vi "mainGenerator.vi"() -> ()   [LabVIEW 2017]
uses:
  Control/states.ctl
  <vilib>/ErrorRing/Error Ring.xnode
  <vilib>/measure/NI_MABase.lvlib
panel:
  out "Sinal":waveform(dbl)(graph)={"t0"=timestamp(0 s since 1904-01-01), "dt"=0.0002, "Y"=[]}
  out "Onda":waveform(dbl)(graph)
  in  "Abrir":bool
  in  "Salvar":bool
  in  "Limpa":bool
  in  "Adicionar":bool
  in  "Configurações\n da Onda":T1={"Tipo de forma de onda "=enum."Sine Wave", "Amplitude "=0.0, "Frequencia "=0.0, "Ciclos "=1.0, "Duty Cycle "=0.0, "% Subida "=0.0, "% High "=0.0, "% Descida "=0.0, "Fase "=0.0, "Offset"=0.0, "% Baixo"=0.0, "Amostragem"=0.0} {"Ciclos" min=1.0; "Frequencia" min=0.0}
  in  "Stop Button":bool
  # "Gerador de Sinais"
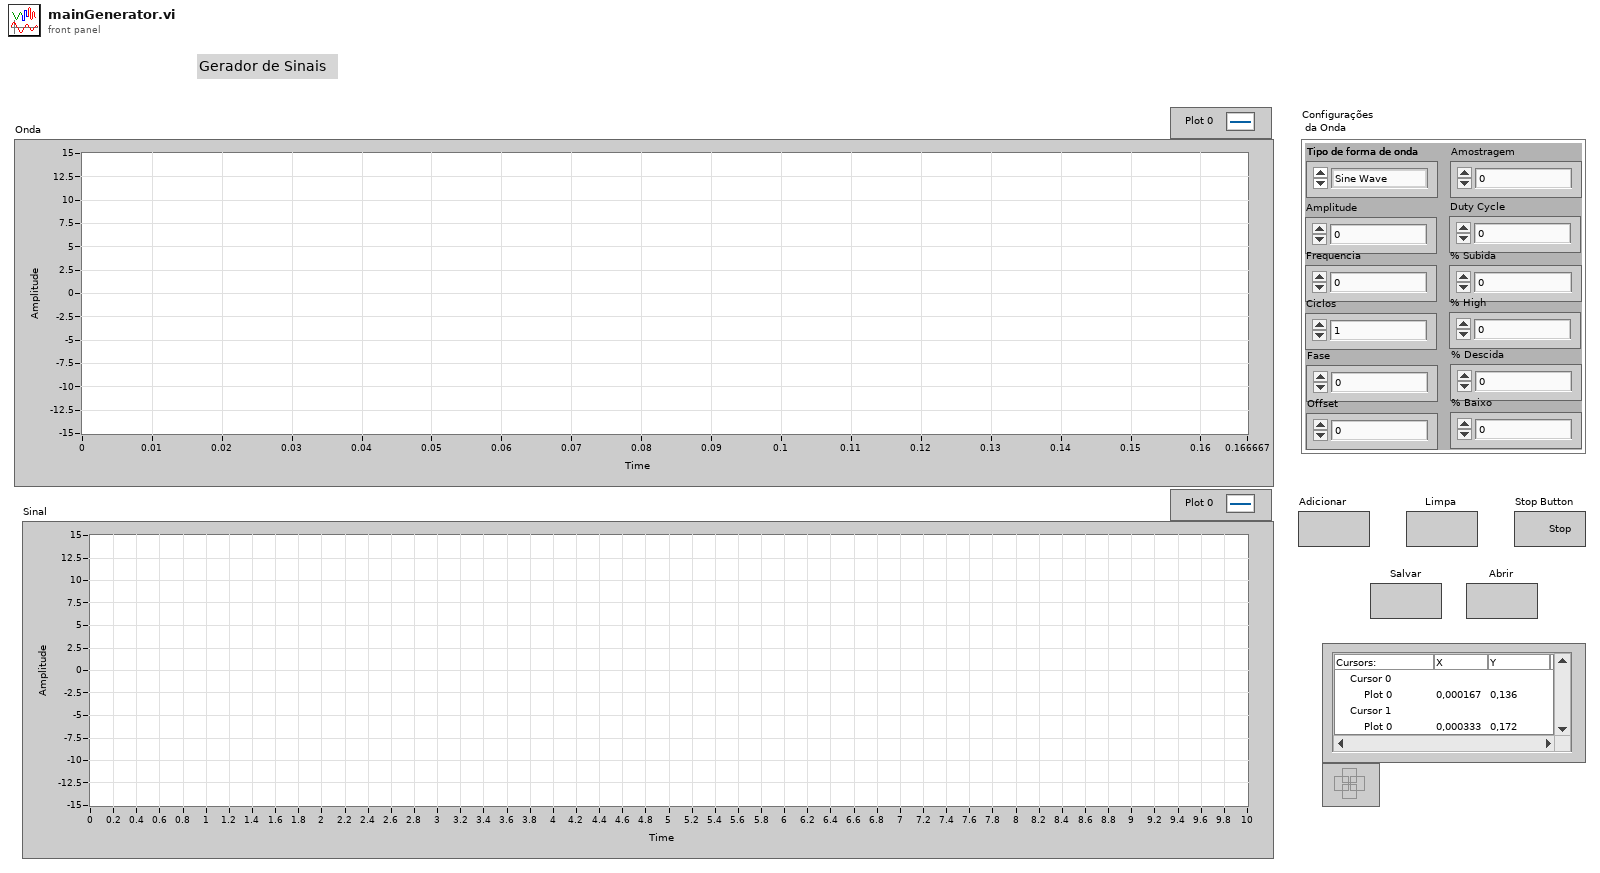
[diagram p1: front panel]
types:
  T1 = cluster{"Tipo de forma de onda ":enum16{"Sine Wave", "Triangle Wave", "Square Wave", "Sawtooth Wave", "Trapezoidal Wave"}, "Amplitude ":dbl, "Frequencia ":dbl, "Ciclos ":dbl, "Duty Cycle ":dbl, "% Subida ":dbl, "% High ":dbl, "% Descida ":dbl, "Fase ":dbl, "Offset":dbl, "% Baixo":dbl, "Amostragem":dbl}
  T2 = typedef "states.ctl" = enum16{"Initialize", "Esperar evento", "Desenha Onda", "Mostra Onda", "Desenha Sinal", "Mostra Sinal", "Clean Graph", "Add", "Remove", "Save", "Open", "Stop"}
  T3 = enum16{"open", "open or create", "create or replace", "create", "open (read-only)"}
  T4 = enum16{"Sine Wave", "Triangle Wave", "Square Wave", "Sawtooth Wave", "Trapezoidal Wave"}
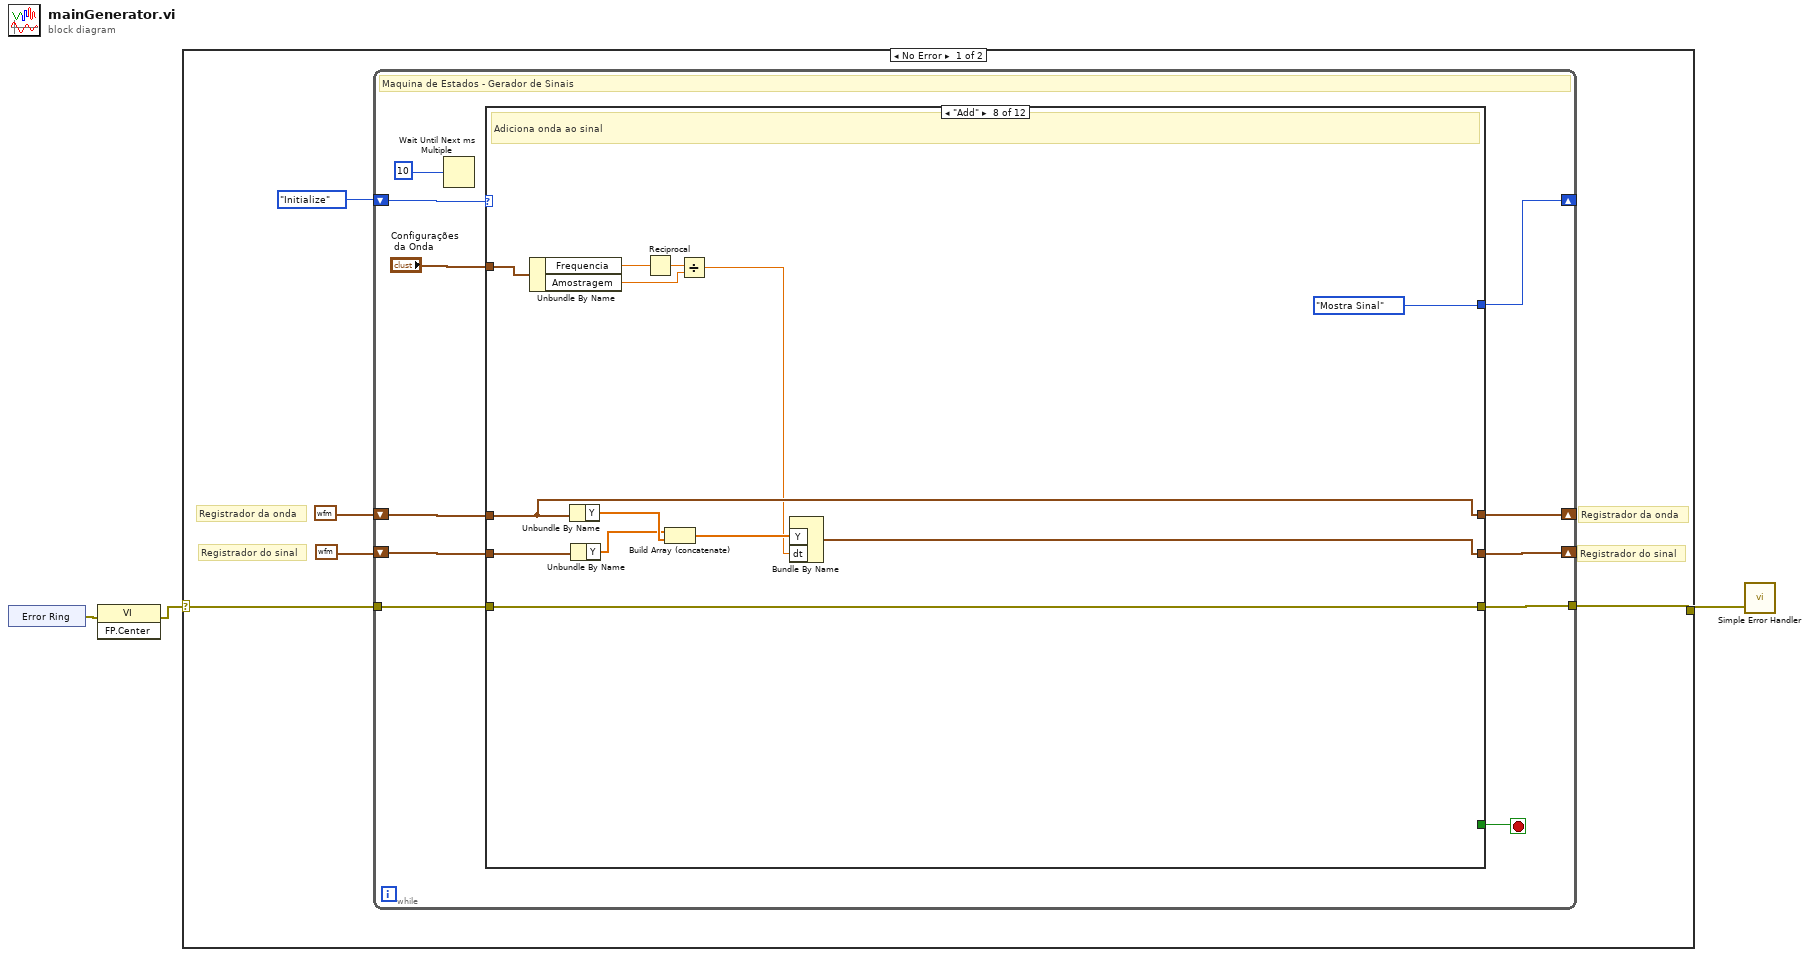
[diagram p0: block diagram]
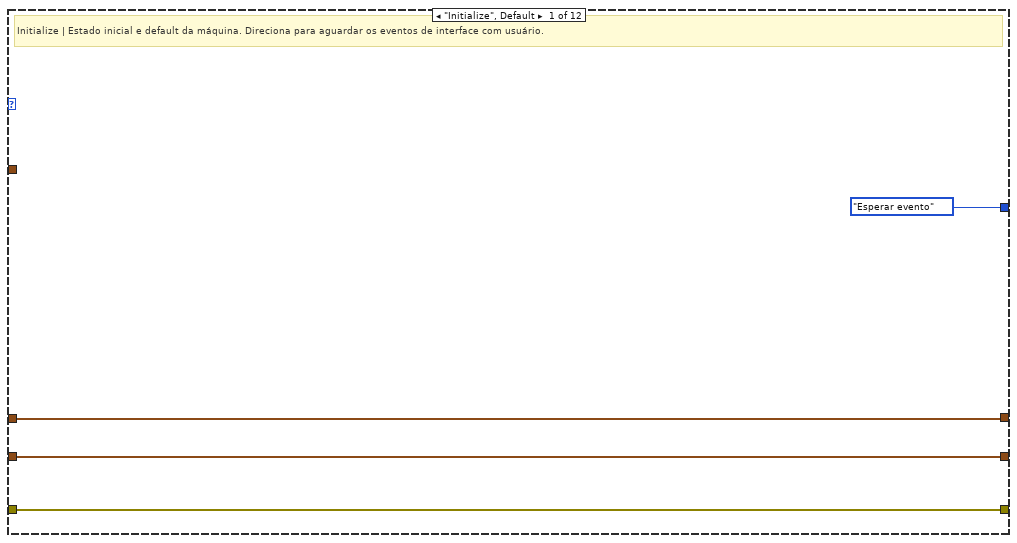
[diagram p2: hidden frame]
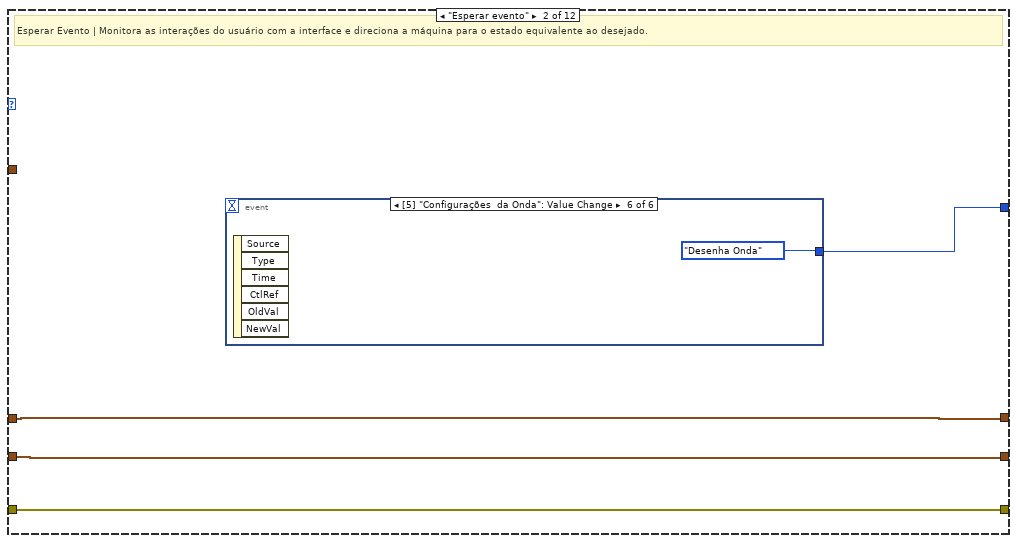
[diagram p3: hidden frame]
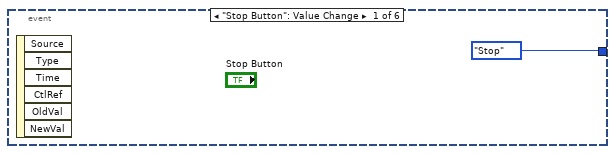
[diagram p4: hidden frame]
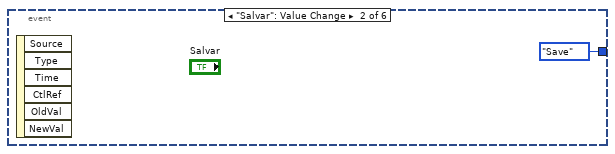
[diagram p5: hidden frame]
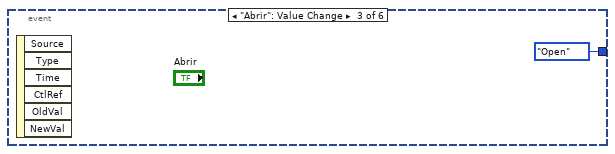
[diagram p6: hidden frame]
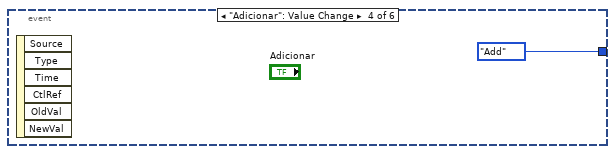
[diagram p7: hidden frame]
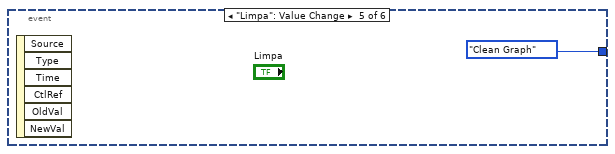
[diagram p8: hidden frame]
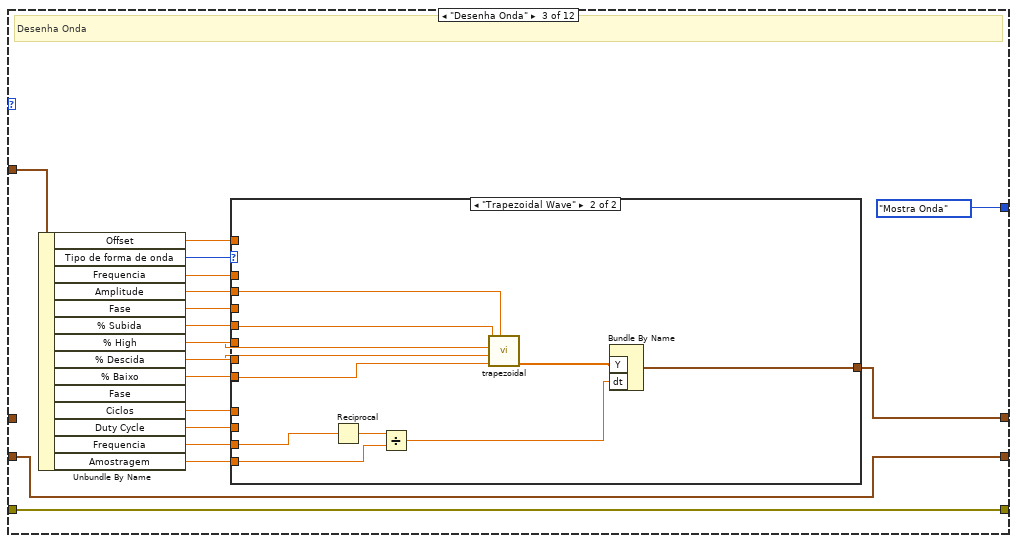
[diagram p9: hidden frame]
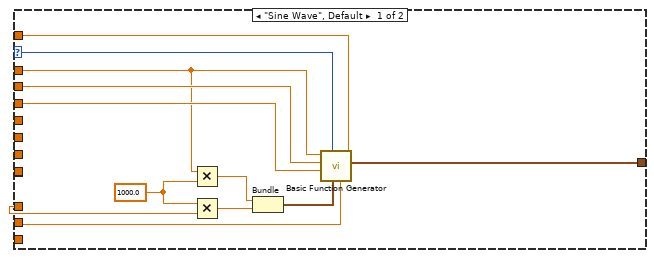
[diagram p10: hidden frame]
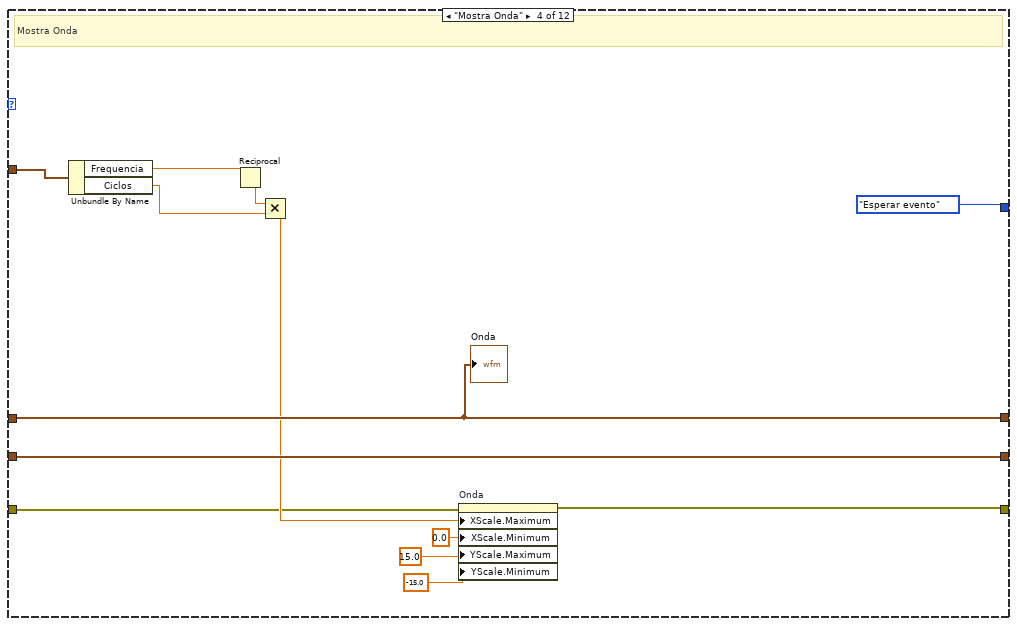
[diagram p11: hidden frame]
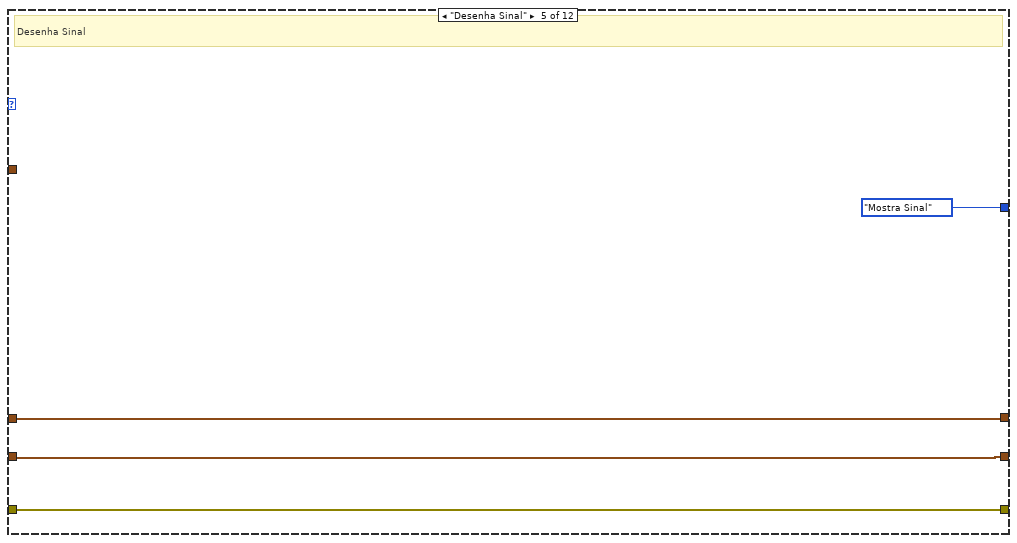
[diagram p12: hidden frame]
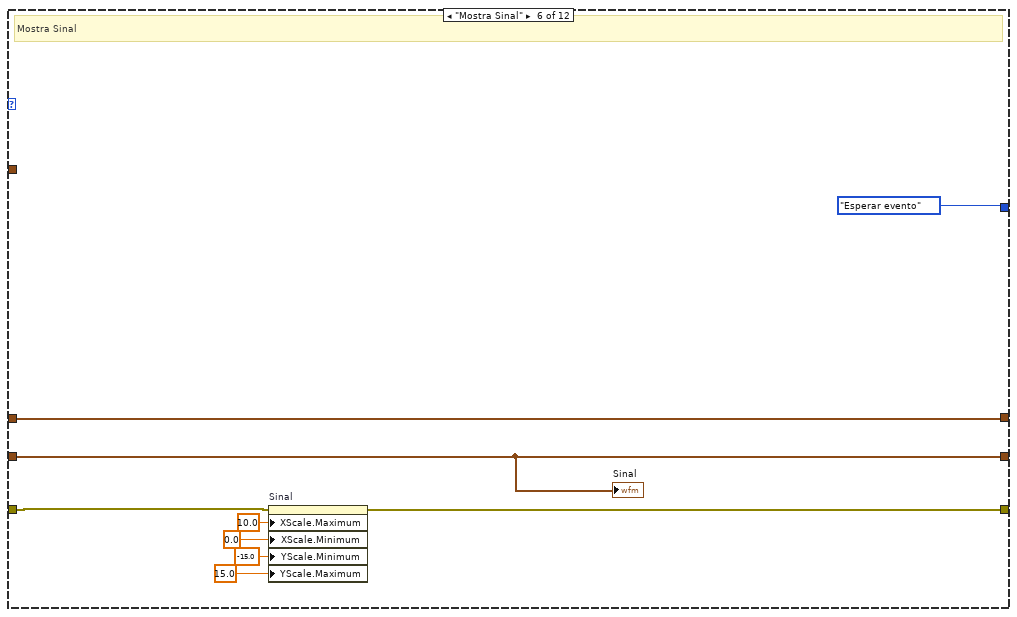
[diagram p13: hidden frame]
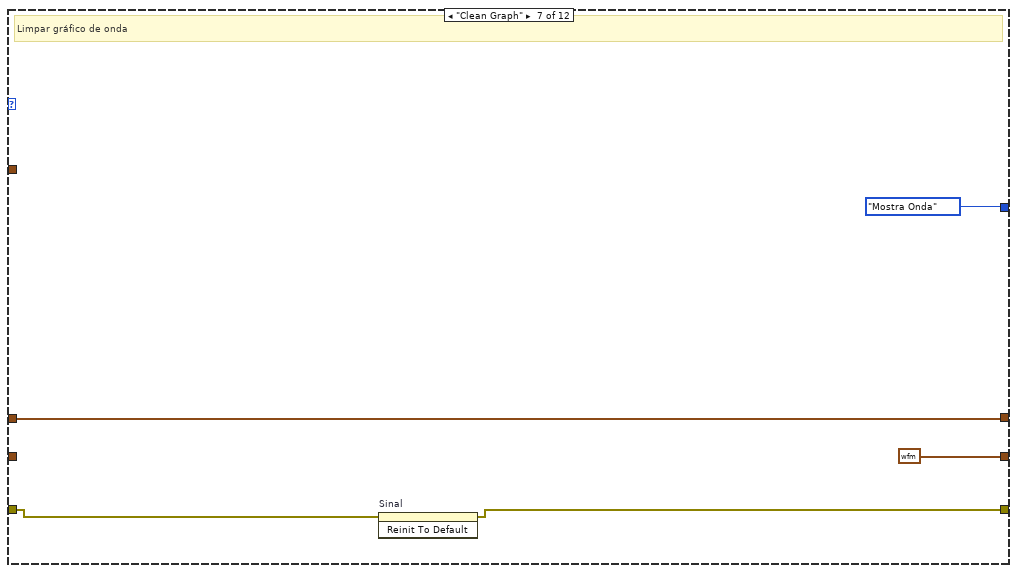
[diagram p14: hidden frame]
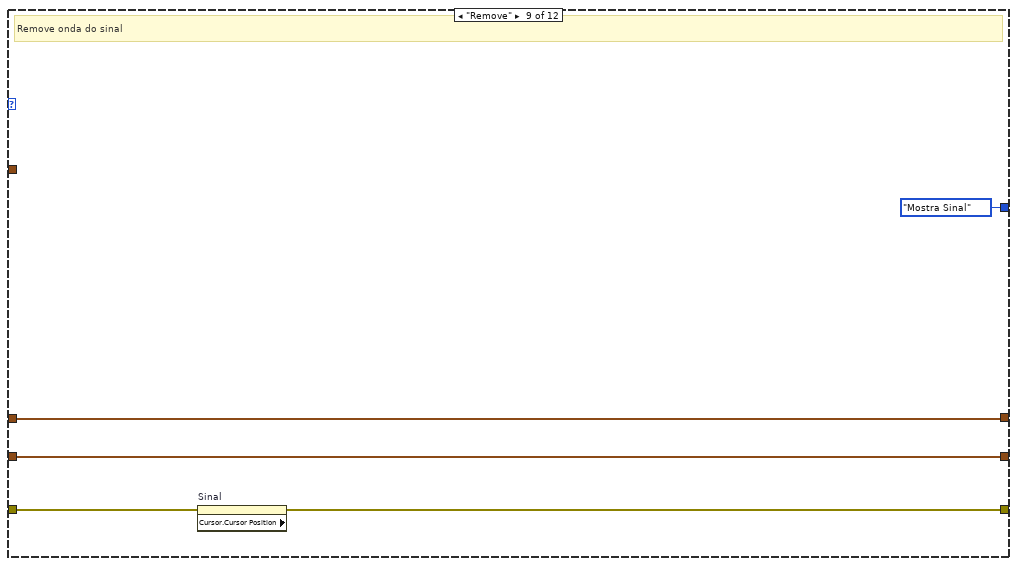
[diagram p15: hidden frame]
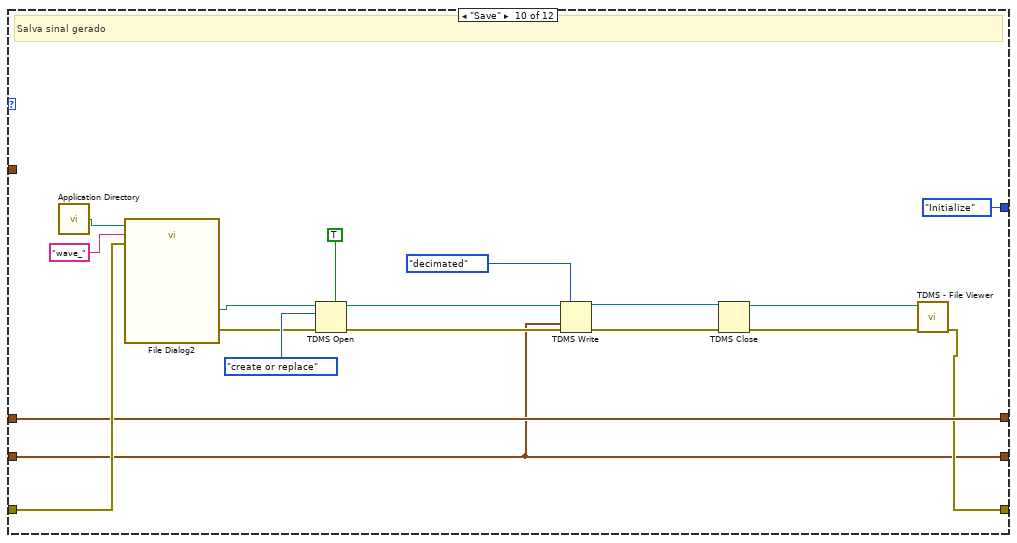
[diagram p16: hidden frame]
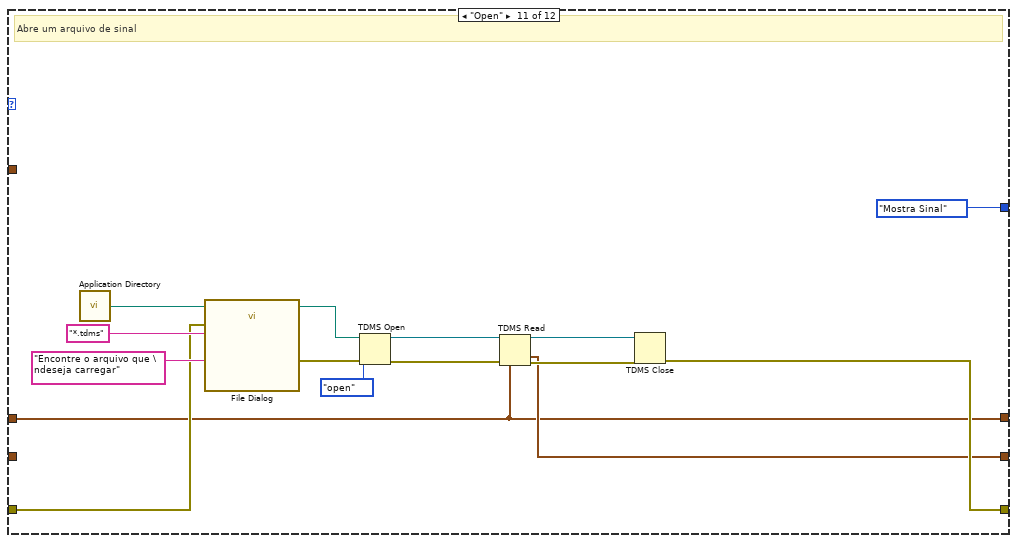
[diagram p17: hidden frame]
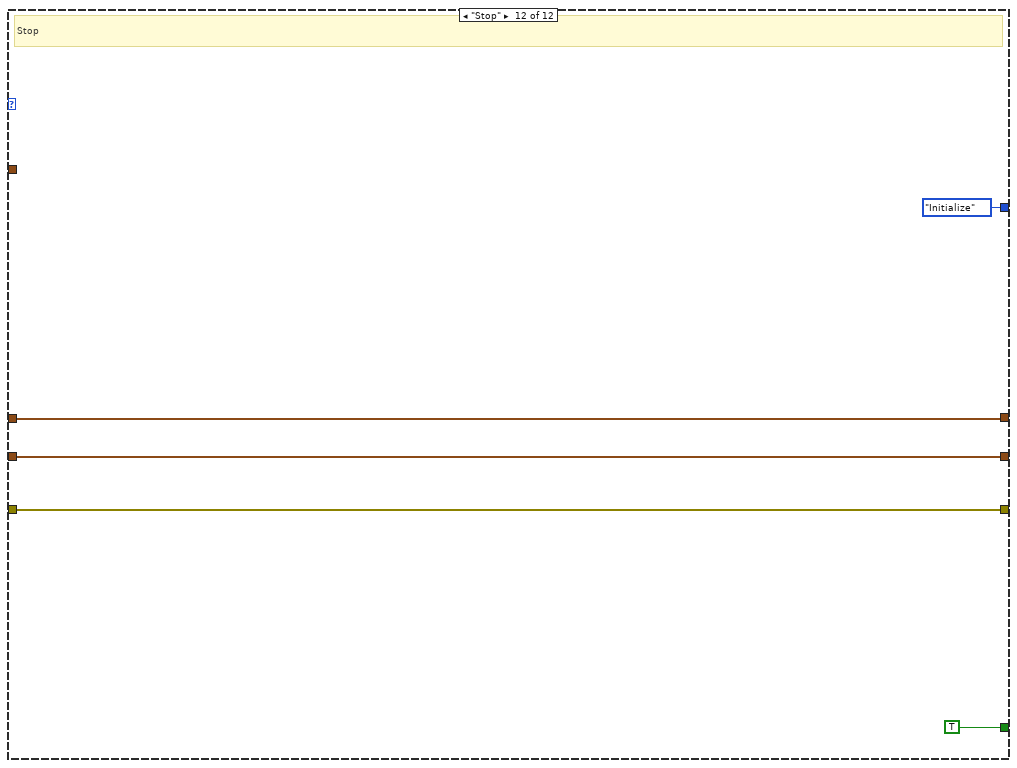
[diagram p18: hidden frame]
diagram:
  n1 = xnode "Error Ring"() -> ("error out"=w3:errorcluster)
  n2 = invoke class="VI" method="FP.Center"(error in=w3) -> (error out=w2:errorcluster)  [unwired: 2 in, 2 out]
  n3 = case shown="No Error" w2 {
    selector: w2 -> [w8 w162]
    tunnel: [w7 w162] -> w1
    frame No Error {
      # "Registrador do sinal"
      # "Registrador da onda"
      # "Registrador do sinal"
      # "Registrador da onda"
      n4 = while {
        shift-right: [w11] -> _
        shift-left: states."Initialize" ("Enum") -> [w12]
        shift-right: [w10] -> _
        shift-left: waveform(dbl) {"t0"=timestamp(0 s since 1904-01-01), "dt"=1.0, "Y"=[]} ("signal out") -> [w13]
        tunnel: [w17] -> w7
        tunnel: w8 -> [w16]
        shift-right: [w14] -> _
        shift-left: waveform(dbl) {"t0"=timestamp(0 s since 1904-01-01), "dt"=1.0, "Y"=[]} ("signal out") -> [w15]
        stop <- w18 stop-if-true
        # "Maquina de Estados - Gerador de Sinais"
        n5 = Wait Until Next ms Multiple(millisecond multiple=u32 10) -> ()  [unwired: 1 out]
        n6 = case shown="\"Add\"" w12 {
          tunnel: [states."Esperar evento" w27 states."Mostra Onda" ("Enum") states."Esperar evento" ("Enum") states."Mostra Sinal" states."Esperar evento" ("Enum") states."Mostra Onda" ("Enum") states."Mostra Sinal" ("Enum") states."Mostra Sinal" ("Enum") states."Initialize" ("Enum") states."Mostra Sinal" ("Enum") states."Initialize" ("Enum")] -> w11
          tunnel: [_ _ _ _ _ _ _ _ _ _ _ TRUE] -> w18
          tunnel: [w21 w24 w37 w83 w90 w100 w104 w108 w122 w128 w142 w161] -> w10
          tunnel: w13 -> [w21 w24 _ w83 w90 w100 w104 w108 w122 w128 w142 w161]
          tunnel: [w23 w26 w35 w75 w91 w92 w101 w107 w119 w125 w146 w160] -> w17
          tunnel: w16 -> [w23 w26 w35 w76 w91 w93 w102 w107 w120 w136 w153 w160]
          tunnel: w15 -> [w22 w25 w41 w87 w88 w98 _ w113 w123 w124 _ w159]
          tunnel: [w22 w25 w41 w87 w88 w98 waveform(dbl) {"t0"=timestamp(0 s since 1904-01-01), "dt"=1.0, "Y"=[]} ("signal out") w109 w123 w124 w143 w159] -> w14
          tunnel: "Configurações\n da Onda" -> [_ _ w39 w85 _ _ _ w117 _ _ _ _]
          frame "Initialize", Default {
            # "Initialize | Estado inicial e default da máquina. Direciona para aguardar os eventos de interface com usuário."
          }
          frame "Esperar evento" {
            # "Esperar Evento | Monitora as interações do usuário com a interface e direciona a máquina para o estado equivalente ao desejado."
            n7 = event shown="[5] \"Configurações  da Onda\": Value Change" {
              selector: _ -> [_ _ _ _ _ _]
              dyn-events: _ -> [_ _ _ _ _ _]
              timeout: _ -> [_ _ _ _ _ _]
              tunnel: [states."Stop" ("Enum") states."Save" ("Enum") states."Open" ("Enum") states."Add" ("Enum") states."Clean Graph" ("Enum") states."Desenha Onda" ("Enum")] -> w27
              event "Stop Button": Value Change {
                n8 = event-data() -> ()  [unwired: 1 in, 6 out]
              }
              event "Salvar": Value Change {
                n9 = event-data() -> ()  [unwired: 1 in, 6 out]
              }
              event "Abrir": Value Change {
                n10 = event-data() -> ()  [unwired: 1 in, 6 out]
              }
              event "Adicionar": Value Change {
                n11 = event-data() -> ()  [unwired: 1 in, 6 out]
              }
              event "Limpa": Value Change {
                n12 = event-data() -> ()  [unwired: 1 in, 6 out]
              }
              event "Configurações\n da Onda": Value Change {
                n13 = event-data() -> ()  [unwired: 1 in, 6 out]
              }
            }
          }
          frame "Desenha Onda" {
            # "Desenha Onda"
            n14 = Unbundle By Name(w39) -> ("Offset"=w47:dbl, "Tipo de forma de onda"=w51:T4, "Frequencia"=w38:dbl, "Amplitude"=w50:dbl, "Fase"=w49:dbl, "% Subida"=w46:dbl, "% High"=w45:dbl, "% Descida"=w44:dbl, "% Baixo"=w43:dbl, "Ciclos"=w36:dbl, "Duty Cycle"=w48:dbl, "Frequencia"=w42:dbl, "Amostragem"=w34:dbl)  [unwired: 1 out]
            n15 = case shown="\"Trapezoidal Wave\"" w51 {
              selector: w51 -> [w63 _]
              tunnel: w38 -> [w56 _]
              tunnel: w50 -> [w62 w74]
              tunnel: w49 -> [w60 _]
              tunnel: w48 -> [w59 _]
              tunnel: w47 -> [w55 _]
              tunnel: w36 -> [w54 _]
              tunnel: [w53 w68] -> w37
              tunnel: w46 -> [_ w73]
              tunnel: w45 -> [_ w72]
              tunnel: w44 -> [_ w71]
              tunnel: [_ w70] -> _
              tunnel: w43 -> [_ w70]
              tunnel: w42 -> [_ w67]
              tunnel: w34 -> [_ w65]
              frame "Sine Wave", Default {
                w52 = 1000.0 ("y")
                n16 = Multiply(x=w56, y=w52) -> (x*y=w57:dbl)
                n17 = Multiply(x=w52, y=w54) -> (x*y=w58:dbl)
                n18 = Bundle(w57, w58) -> (w61:cluster{dbl, dbl})  [unwired: 1 in]
                n19 = call <vilib>:"Basic Function Generator.vi"("offset"=w55, "square wave duty cycle (%)"=w59, "sampling info"=w61, "signal type"=w63, "phase"=w60, "amplitude"=w62, "frequency"=w56) -> ("signal out"=w53:waveform(dbl))  [unwired: 2 in, 2 out]
              }
              frame "Trapezoidal Wave" {
                n20 = Reciprocal(x=w67) -> (1/x=w66:dbl)
                n21 = Divide(x=w66, y=w65) -> (x/y=w64:dbl)
                n22 = call "trapezoidal.vi"("%Subida"=w73, "%Alto"=w72, "%Descida"=w71, "%Baixo"=w70, "Amplitude"=w74) -> ("Waveform Graph"=w69:dbl[])  [unwired: 5 in]
                n23 = Bundle By Name("Y"=w69, "dt"=w64) -> (w68:waveform(dbl))  [unwired: 1 in]
              }
            }
          }
          frame "Mostra Onda" {
            # "Mostra Onda"
            n24 = Unbundle By Name(w85) -> ("Frequencia"=w84:dbl, "Ciclos"=w81:dbl)
            n25 = Reciprocal(x=w84) -> (1/x=w82:dbl)
            n26 = Multiply(x=w82, y=w81) -> (x*y=w80:dbl)
            n27 = property on="Onda" class="WFGraph (strict)"(error in=w76, "XScale.Maximum"=w80, "XScale.Minimum"=0.0 ("X Scale.Range:Minimum"), "YScale.Maximum"=15.0 ("Y Scale.Range:Maximum"), "YScale.Minimum"=-15.0 ("Y Scale.Range:Minimum")) -> (error out=w75:errorcluster)  [unwired: 1 in, 1 out]
            "Onda" <- w83
          }
          frame "Desenha Sinal" {
            # "Desenha Sinal"
          }
          frame "Mostra Sinal" {
            # "Mostra Sinal"
            n28 = property on="Sinal" class="WFGraph (strict)"(error in=w93, "XScale.Maximum"=10.0 ("X Scale.Range:Maximum"), "XScale.Minimum"=0.0 ("X Scale.Range:Minimum"), "YScale.Minimum"=-15.0 ("Y Scale.Range:Minimum"), "YScale.Maximum"=15.0 ("Y Scale.Range:Maximum")) -> (error out=w92:errorcluster)  [unwired: 1 in, 1 out]
            "Sinal" <- w98
          }
          frame "Clean Graph" {
            # "Limpar gráfico de onda"
            n29 = invoke on="Sinal" class="WFGraph (strict)" method="Reinit To Default"(error in=w102) -> (error out=w101:errorcluster)  [unwired: 2 in, 2 out]
          }
          frame "Add" {
            # "Adiciona onda ao sinal"
            n30 = Unbundle By Name(w117) -> ("Frequencia"=w116:dbl, "Amostragem"=w114:dbl)
            n31 = Unbundle By Name(w108) -> ("Y"=w112:dbl[])
            n32 = Unbundle By Name(w113) -> ("Y"=w111:dbl[])
            n33 = Reciprocal(x=w116) -> (1/x=w115:dbl)
            n34 = Build Array (concatenate)(w111, w112) -> (w110:dbl[])
            n35 = Divide(x=w115, y=w114) -> (x/y=w106:dbl)
            n36 = Bundle By Name("Y"=w110, "dt"=w106) -> (w109:waveform(dbl))  [unwired: 1 in]
          }
          frame "Remove" {
            # "Remove onda do sinal"
            n37 = property on="Sinal" class="WFGraph (strict)" props=["Cursor", "Cursor Position"](error in=w120) -> (error out=w119:errorcluster)  [unwired: 1 in, 2 out]
          }
          frame "Save" {
            # "Salva sinal gerado"
            n38 = call <vilib>:"Application Directory.vi"() -> ("Application Directory"=w133:path)
            n39 = call "File Dialog2"("start path"=w133, "default name"="wave_", "error in"=w136) -> ("selected path"=w134:path, "error out"=w135:errorcluster)  [unwired: 9 in, 2 out]
            n40 = TDMS Open(5:TRUE ("create index file? (T)"), 8:w135, 10:T3."create or replace" ("operation (0:open)"), 11:w134) -> (0:w129:errorcluster, 3:w130:refnum<k34>)  [unwired: 3 in]
            n41 = TDMS Write(0:w130, 1:enum16{"decimated", "interleaved"}."decimated" ("data layout (0:decimated)"), 9:w124, 11:w129) -> (4:w141:refnum<k34>, 15:w140:errorcluster)  [unwired: 2 in, 2 out]
            n42 = TDMS Close(8:w140, 11:w141) -> (0:w126:errorcluster, 3:w127:path)
            n43 = call <vilib>:"TDMS - File Viewer.vi"("error in (no error)"=w126, "file path"=w127) -> ("error out"=w125:errorcluster)  [unwired: 4 in, 1 out]
          }
          frame "Open" {
            # "Abre um arquivo de sinal"
            n44 = call <vilib>:"Application Directory.vi"() -> ("Application Directory"=w156:path)
            n45 = call "File Dialog"("start path"=w156, "prompt"="Encontre o arquivo que \ndeseja carregar", "error in"=w153, "pattern (all files)"="*.tdms") -> ("selected path"=w151:path, "error out"=w152:errorcluster)  [unwired: 8 in, 2 out]
            n46 = TDMS Open(8:w152, 10:T3."open" ("operation (0:open)"), 11:w151) -> (0:w149:errorcluster, 3:w148:refnum<k34>)  [unwired: 4 in]
            n47 = TDMS Read(0:w148, 11:w149, 12:w142) -> (4:w145:refnum<k34>, 10:w143:waveform(dbl), 15:w147:errorcluster)  [unwired: 5 in, 3 out]
            n48 = TDMS Close(8:w147, 11:w145) -> (0:w146:errorcluster)  [unwired: 1 out]
          }
          frame "Stop" {
            # "Stop"
          }
        }
      }
    }
    frame Error {
    }
  }
  n49 = call <vilib>:"Simple Error Handler.vi"("error in (no error)"=w1) -> ()  [unwired: 4 in, 5 out]
